vi "2s Complement to Decimal.vi"(11 "2s Complement In":u16) -> (3 "Decimal Number Out":dbl format="%.2f")   [LabVIEW 2019]
doc: "Converts a 12-bit 2s complement to a DBL decimal number."
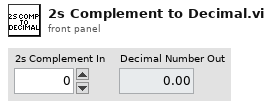
[diagram p1: front panel]
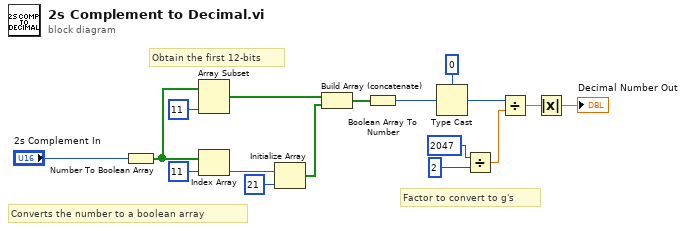
[diagram p0: block diagram]
diagram:
  # "Converts the number to a boolean array"
  # "Obtain the first 12-bits"
  # "Factor to convert to g's"
  n1 = Number To Boolean Array(number="2s Complement In") -> (Boolean array=w17:bool[])
  n2 = Array Subset(array=w17, length=11 ("index")) -> (w12:bool[])  [unwired: 1 in]
  n3 = Index Array(array=w17, index=11) -> (element=w13:bool)
  n4 = Initialize Array(w13, 21 ("dimension size")) -> (w11:bool[])
  n5 = Build Array (concatenate)(w12, w11) -> (w10:bool[])
  n6 = Boolean Array To Number(Boolean array=w10) -> (number=w9:u32)
  n7 = Type Cast(type=0 ("dimension size"), x=w9) -> (*(type *) &x=w1:i32)
  n8 = Divide(x=u16 2047 ("A_X (g)"), y=u16 2) -> (x/y=w5:dbl)
  n9 = Divide(x=w1, y=w5) -> (x/y=w4:dbl)
  n10 = Absolute Value(x=w4) -> (abs(x)=→"Decimal Number Out":dbl)
